vi "read.vi"(6 "timeout ms (1000)":i32=1000, 8 "error in":errorcluster, 11 "TCP in":refnum<k5>) -> (0 "error out":errorcluster, 1 "Timeout":bool, 2 "Read Data Cluster":T1, 3 "TCP out":refnum<k5>)   [LabVIEW 2025, in "Newtons4thEkg.lvlib"]
uses:
  Newtons4thEkg.lvlib
  Typedefs/ReadData.ctl
  <vilib>/Platform/TimedLoop/XDataNode/timing_clust.ctl
  <vilib>/Platform/TimedLoop/XDataNode/nitl_modes.ctl
  <vilib>/Platform/TimedLoop/XDataNode/wakeup.ctl
  <vilib>/platform/TimedLoop/XDataNode/XDataNode.xnode
  <vilib>/Platform/TimedLoop/XDataNode/XDNodeRunTimeDep.lvlib
panel:
  out "Identificaton":string="192.168.0.28"
  in  "IP Address":string="192.168.1.101"
  in  "Initialize":bool
  out "Response [ms]":dbl format="%.1f"
  in  "Period [ms]":i32=500 min=1 max=60000
  in  "Read Continuous":bool
  # "Driver Testing"
  # "note: Measurement window is set to MEDUIM (0.33 s), which is sufficient for 0.5 measurement including TCP latency. When a timeout occurs, the driver returns NaN.  \nTimeout error may appear when frequency is synchronizing. Timeout is cleared and indicated as boolean output."
  # "Newtons4th V0.10\nRead"
  # "05.05.2025"
  # "Blaz Kelbl"
  # "Newtons4th V0.10\nRead"
  # "05.05.2025"
  # "Blaz Kelbl"
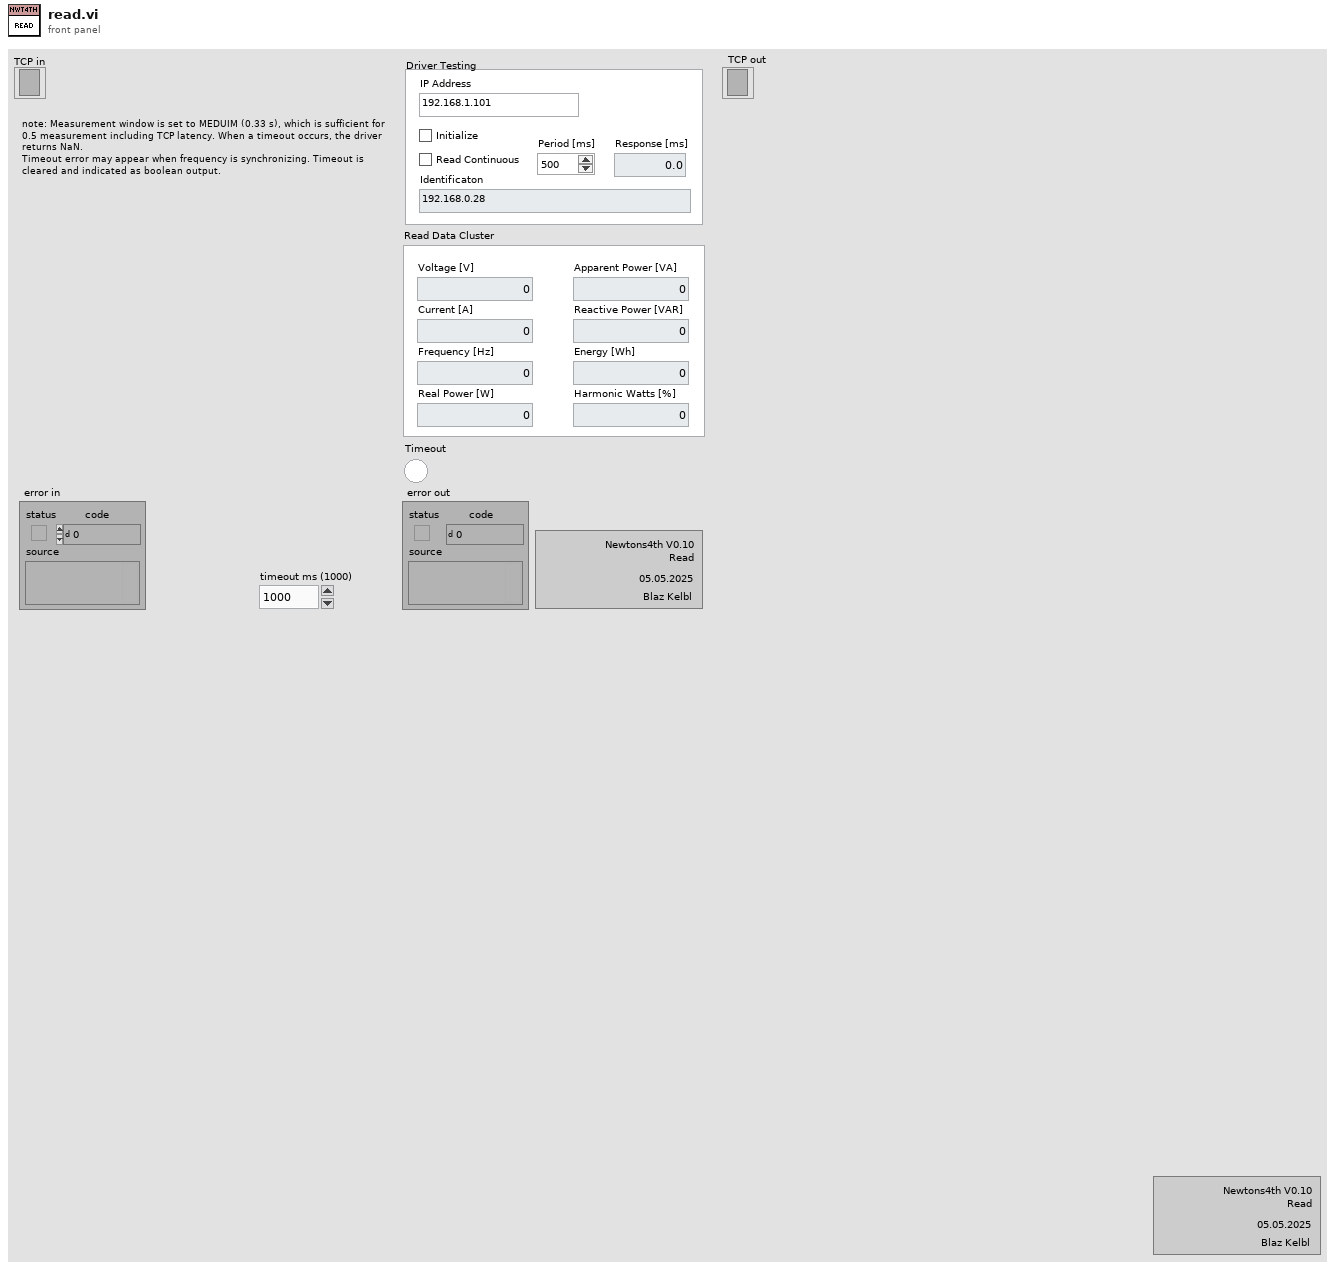
[diagram p1: front panel]
types:
  T1 = typedef "Newtons4thEkg.lvlib/ReadData.ctl" = cluster{"Voltage [V]":dbl, "Current [A]":dbl, "Frequency [Hz]":dbl, "Real Power [W]":dbl, "Apparent Power [VA]":dbl, "Reactive Power [VAR]":dbl, "Energy [Wh]":dbl, "Harmonic Watts [%]":dbl}
  T2 = typedef "XDNodeRunTimeDep.lvlib/timing_clust.ctl" = cluster{"Expected End [f-1]":u64, "Actual End [f-1]":u64, "Finished Late? [f-1]":bool, "Expected End [i-1]":u64, "Actual End [i-1]":u64, "Finished Late? [i-1]":bool, "Expected Start [i]":u64, "Actual Start [i]":u64, "Expected Start [f]":u64, "Actual Start [f]":u64, "Source Name":string, "Structure Name":string, "Period":i64, "Deadline":i64, "Offset":i64, "Start":i64, "Priority":i32, "Timeout":i32, "Mode":T3, "Wakeup Reason":T4, "Error":errorcluster, "Source Type":string, "Secondary Source Type":string, "Global End Time":u64, "Global Start Time":u64, "Frame Duration":u64, "Iteration Duration":u64, "Assigned CPU":i32, "I/O Scan Engine Mode":u32}
  T3 = typedef "XDNodeRunTimeDep.lvlib/nitl_modes.ctl" = enum32{"No Change", "Process missed periods, maintain original phase", "Discard missed periods, maintain original phase", "Process missed periods, ignore original phase", "Discard missed periods, ignore original phase"}
  T4 = typedef "XDNodeRunTimeDep.lvlib/wakeup.ctl" = enum32{"Normal", "Aborted", "Asynchronous wakeup", "Timing source error", "Timed loop error", "Timeout"}
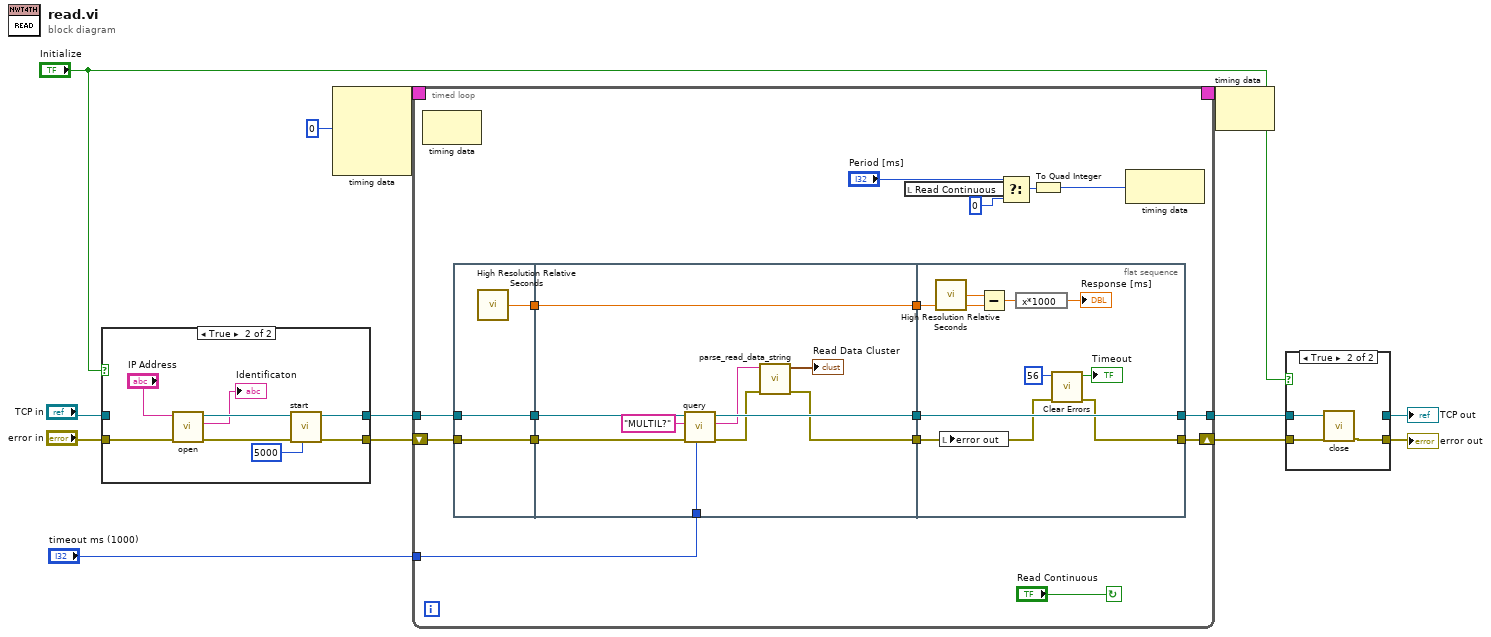
[diagram p0: block diagram]
diagram:
  n1 = case shown="True" "Initialize" {
    tunnel: "error in" -> [w14 w22]
    tunnel: [w14 w18] -> w9
    tunnel: [w15 w19] -> w8
    tunnel: "TCP in" -> [w15 _]
    frame False {
    }
    frame True {
      n2 = call "open.vi"("error in"=w22, "IP Address"="IP Address") -> ("error out"=w21:errorcluster, "Identification"=→"Identificaton":string, "TCP"=w20:refnum<k5>)  [unwired: 7 in]
      n3 = call "start.vi"("timeout ms (1000)"=5000, "error in (no error)"=w21, "TCP Network Connection in"=w20) -> ("error out"=w18:errorcluster, "TCP Network Connection out"=w19:refnum<k5>)  [unwired: 6 in, 1 out]
    }
  }
  n4 = node-c288(i64 0 ("Period")) -> (w13:T2)  [unwired: 3 in]
  n5 = timed-loop {
    timing: w13 -> [_]
    timing-out: [_] -> w12
    tunnel: w8 -> [w36]
    tunnel: [w35] -> w6
    shift-right: [w31] -> w5
    shift-left: w9 -> [w34]
    tunnel: "timeout ms (1000)" -> [w26]
    stop <- "Read Continuous" continue-if-true
    n6 = node-c288() -> ()  [unwired: 1 in, 1 out]
    n7 = flat-sequence {
      tunnel: w34 -> [w42]
      tunnel: w36 -> [w43]
      tunnel: [w43] -> w30
      tunnel: [w42] -> w29
      tunnel: [w41] -> w27
      tunnel: [w49] -> w33
      tunnel: [w44] -> w32
      tunnel: w30 -> [w53]
      tunnel: w29 -> [w52]
      tunnel: [w51] -> w28
      tunnel: w27 -> [w51]
      tunnel: w26 -> [w48]
      tunnel: [w56] -> w31
      tunnel: [w62] -> w35
      tunnel: w33 -> [w62]
      tunnel: w32 -> [w61]
      tunnel: w28 -> [w58]
      frame #0 {
        n8 = call <vilib>:"High Resolution Relative Seconds.vi"() -> ("relative seconds"=w41:dbl)
      }
      frame #1 {
        n9 = call "query.vi"("timeout ms (1000)"=w48, "error in (no error)"=w52, "Query"="MULTIL?", "TCP in"=w53) -> ("error out"=w47:errorcluster, "Return String"=w46:string, "TCP out"=w49:refnum<k5>)  [unwired: 5 in]
        n10 = call "parse_read_data_string.vi"("error in"=w47, "Read Data String"=w46) -> ("error out"=w44:errorcluster, "Read Data Cluster"=→"Read Data Cluster":T1)  [unwired: 8 in]
      }
      frame #2 {
        n11 = call <vilib>:"High Resolution Relative Seconds.vi"() -> ("relative seconds"=w60:dbl)
        n12 = local write "error out"(w61) -> ()
        n13 = Subtract(x=w60, y=w58) -> (x-y=w59:dbl)
        n14 = expression code="x*1000"(w59) -> (→"Response [ms]":dbl)
        n15 = call <vilib>:"Clear Errors.vi"("error in (no error)"=w61, "specific error code to clear (0: all)"=56) -> ("error out"=w56:errorcluster, "specific error cleared?"=→"Timeout":bool)  [unwired: 4 in]
      }
    }
    n16 = local read "Read Continuous"() -> (w40:bool)
    n17 = Select(t="Period [ms]", s=w40, f=0) -> (s? t:f=w38:i32)
    n18 = To Quad Integer(1:w38) -> (0:w37:i64)
    n19 = node-c288(w37) -> ()  [unwired: 1 out]
  }
  n20 = node-c288(w12) -> ()  [unwired: 1 out]
  n21 = case shown="True" "Initialize" {
    tunnel: w6 -> [w68 w69]
    tunnel: w5 -> [w67 w71]
    tunnel: [w68 _] -> w4
    tunnel: [w67 w70] -> w3
    frame False {
    }
    frame True {
      n22 = call "close.vi"("error in"=w71, "TCP"=w69) -> ("error out"=w70:errorcluster)  [unwired: 8 in, 1 out]
    }
  }
  "TCP out" <- w4
  "error out" <- w3
